vi "FGV System Konstanten.vi"(6 "Aktionen":T3, 8 "error in":errorcluster caption="error out", 9 "Cluster in":T2, 11 "Sprache":u32) -> (0 "error out":errorcluster, 1 "Cluster out":T1, 2 "LanguageList":string, 3 "Sprachindex":u16, 4 "SysLogLevel":u32)   [LabVIEW 2020, in "System Einstellungen V2.lvlib"]
uses:
  Aktioen FGV System Konstanten.ctl
  <vilib>/Utility/config.llb/Read Key (String).vi
  <vilib>/Utility/config.llb/Read Key (U32).vi
  <vilib>/Utility/config.llb/Write Key (String).vi
  <vilib>/Utility/config.llb/Write Key (U32).vi
  System Einstellungen V2.lvlib
  <vilib>/Utility/config.llb/NI_LVConfig.lvlib
  Allgemein/allgemeine Sub-VIs.lvlib
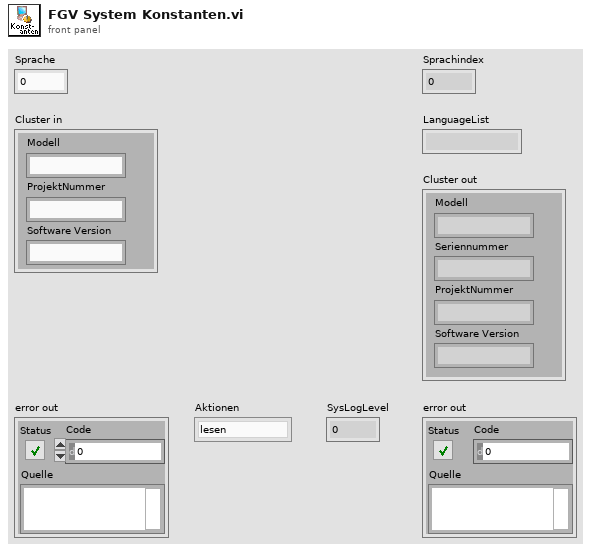
[diagram p1: front panel]
types:
  T1 = cluster{"Modell":string, "ProjektNummer":string, "Software Version":string, "Seriennummer":string}
  T2 = cluster{"Modell":string, "ProjektNummer":string, "Software Version":string}
  T3 = typedef "System Einstellungen V2.lvlib/Aktioen FGV System Konstanten.ctl" = enum16{"lesen", "laden", "speichern", "Sprache"}
  T4 = typedef "NI_LVConfig.lvlib/Config Data RefNum.ctl" = refnum<k1>
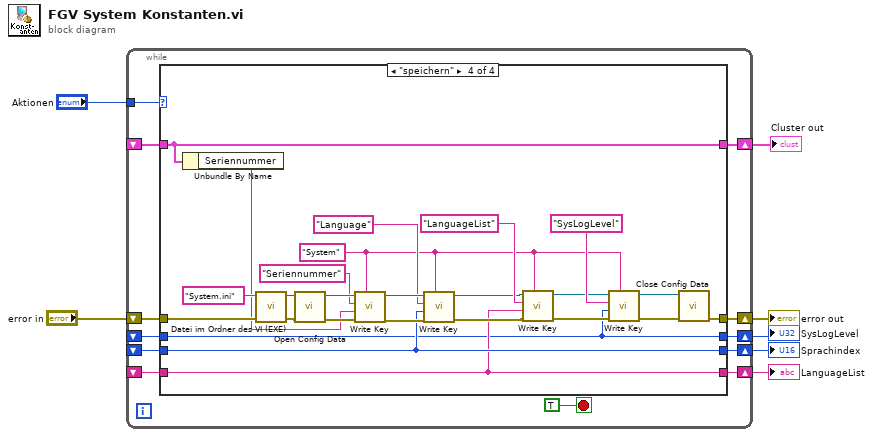
[diagram p0: block diagram]
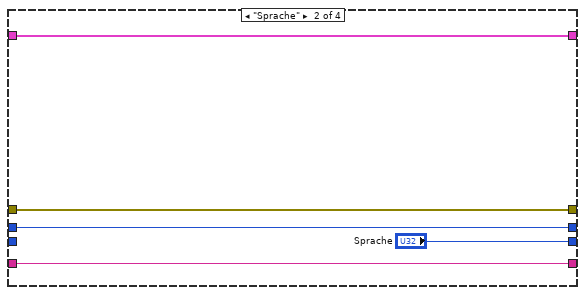
[diagram p3: hidden frame]
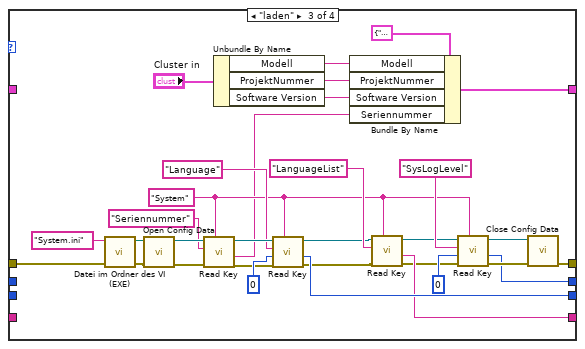
[diagram p4: hidden frame]
diagram:
  n1 = while {
    tunnel: "Aktionen" -> [w18]
    shift-right: [w17] -> w6
    shift-left: _ -> [w16]
    shift-right: [w15] -> w5
    shift-left: _ -> [w14]
    shift-right: [w13] -> w4
    shift-left: "error in" -> [w12]
    shift-right: [w11] -> w2
    shift-left: _ -> [w10]
    shift-right: [w9] -> w1
    shift-left: _ -> [w8]
    stop <- TRUE stop-if-true
    n2 = case shown="\"speichern\"" w18 {
      tunnel: [w24 "Sprache" w52 w64] -> w17
      tunnel: w16 -> [w24 _ _ w64]
      tunnel: [w23 w28 w47 w63] -> w15
      tunnel: w14 -> [w23 w28 _ w63]
      tunnel: [w22 w27 w41 w69] -> w13
      tunnel: w12 -> [w22 w27 w38 w66]
      tunnel: [w21 w26 w37 w62] -> w11
      tunnel: w10 -> [w21 w26 _ w62]
      tunnel: [w20 w25 w31 w61] -> w9
      tunnel: w8 -> [w20 w25 _ w61]
      frame "lesen", Default {
      }
      frame "Sprache" {
      }
      frame "laden" {
        w44 = "System" ("section")
        n3 = call "Datei im Ordner des VI (EXE).vi"("Dateiname"="System.ini") -> ("Dateipfad im Ordner des Haupt-VIs"=w59:path)  [unwired: 8 in, 2 out]
        n4 = call <vilib>:"Open Config Data.vi"("error in (no error)"=w38, "configuration file path"=w59) -> ("error out"=w57:errorcluster, "refnum"=w58:T4)  [unwired: 7 in, 1 out]
        n5 = call-poly <vilib>:"Read Key.vi"("section"=w44, "error in (no error)"=w57, "key"="Seriennummer", "refnum"=w58) -> ("error out"=w51:errorcluster, "value"=w30:string, "refnum out"=w55:T4)  [unwired: 4 in, 1 out]
        n6 = Unbundle By Name("Cluster in") -> ("Modell"=w35:string, "ProjektNummer"=w34:string, "Software Version"=w32:string)
        n7 = call-poly <vilib>:"Read Key.vi"("section"=w44, "error in (no error)"=w51, "default value"=u16 0, "key"="Language" ("section"), "refnum"=w55) -> ("error out"=w48:errorcluster, "value"=w52:u32, "refnum out"=w49:T4)  [unwired: 3 in, 1 out]
        n8 = Bundle By Name(cluster=T1 {"Modell"="", "ProjektNummer"="", "Software Version"="", "Seriennummer"=""} ("Cluster out"), "Modell"=w35, "ProjektNummer"=w34, "Software Version"=w32, "Seriennummer"=w30) -> (w31:T1)
        n9 = call-poly <vilib>:"Read Key.vi"("section"=w44, "error in (no error)"=w48, "key"="LanguageList", "refnum"=w49) -> ("error out"=w43:errorcluster, "value"=w47:string, "refnum out"=w40:T4)  [unwired: 4 in, 1 out]
        n10 = call-poly <vilib>:"Read Key.vi"("section"=w44, "error in (no error)"=w43, "default value"=u16 0, "key"="SysLogLevel" ("section"), "refnum"=w40) -> ("error out"=w42:errorcluster, "value"=w37:u32, "refnum out"=w39:T4)  [unwired: 3 in, 1 out]
        n11 = call <vilib>:"Close Config Data.vi"("error in (no error)"=w42, "refnum"=w39) -> ("error out"=w41:errorcluster)  [unwired: 8 in, 1 out]
      }
      frame "speichern" {
        w72 = "System" ("section")
        n12 = Unbundle By Name(w61) -> ("Seriennummer"=w65:string)
        n13 = call "Datei im Ordner des VI (EXE).vi"("Dateiname"="System.ini") -> ("Dateipfad im Ordner des Haupt-VIs"=w83:path)  [unwired: 8 in, 2 out]
        n14 = call <vilib>:"Open Config Data.vi"("error in (no error)"=w66, "configuration file path"=w83) -> ("error out"=w81:errorcluster, "refnum"=w82:T4)  [unwired: 7 in, 1 out]
        n15 = call-poly <vilib>:"Write Key.vi"("section"=w72, "error in (no error)"=w81, "value"=w65, "key"="Seriennummer", "refnum"=w82) -> ("error out"=w77:errorcluster, "refnum out"=w79:T4)  [unwired: 4 in, 1 out]
        n16 = call-poly <vilib>:"Write Key.vi"("section"=w72, "error in (no error)"=w77, "value"=w64, "key"="Language" ("section"), "refnum"=w79) -> ("error out"=w74:errorcluster, "refnum out"=w75:T4)  [unwired: 4 in, 1 out]
        n17 = call-poly <vilib>:"Write Key.vi"("section"=w72, "error in (no error)"=w74, "value"=w63, "key"="LanguageList", "refnum"=w75) -> ("error out"=w71:errorcluster, "refnum out"=w68:T4)  [unwired: 4 in, 1 out]
        n18 = call-poly <vilib>:"Write Key.vi"("section"=w72, "error in (no error)"=w71, "value"=w62, "key"="SysLogLevel" ("section"), "refnum"=w68) -> ("error out"=w70:errorcluster, "refnum out"=w67:T4)  [unwired: 4 in, 1 out]
        n19 = call <vilib>:"Close Config Data.vi"("error in (no error)"=w70, "refnum"=w67) -> ("error out"=w69:errorcluster)  [unwired: 8 in, 1 out]
      }
    }
  }
  "Sprachindex" <- w6
  "LanguageList" <- w5
  "error out" <- w4
  "SysLogLevel" <- w2
  "Cluster out" <- w1
